vi "Send Generate Event.vi"(8 "Error In":errorcluster, 10 "Event":refnum<class "Event.lvclass">, 11 "Event Source Address":refnum<class "Message Enqueuer.lvclass">) -> (0 "Error Out":errorcluster, 3 "Event Source Address Out":refnum<class "Message Enqueuer.lvclass">)   [LabVIEW 2015, in "Event Source.lvlib" / "Generate Event Msg.lvclass"]
doc: "Send a message to the Event Source Actor to generate the specified event. This method should be called from helper loops within actor core of the Event Source Actor. When the Event Source Actor receives this message he will call Generate Event method.\n\nOnly through calling this method in the helper loops you can be sure all registrants are notified."
uses:
  Generate Event Msg.lvclass
  <vilib>/ActorFramework/Message Enqueuer/Message Enqueuer.lvclass
  Event/Event.lvclass
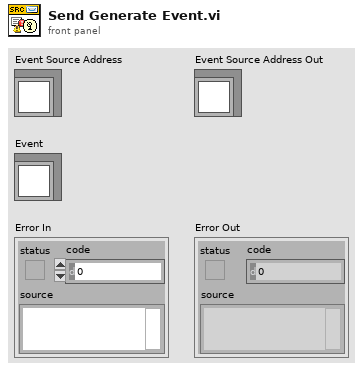
[diagram p1: front panel]
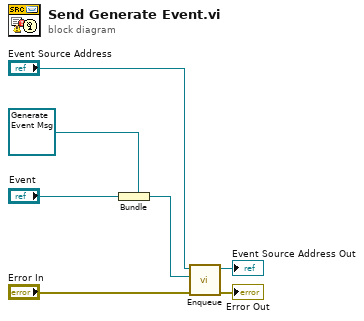
[diagram p0: block diagram]
diagram:
  n1 = Bundle(cluster=refnum<class "Generate Event Msg.lvclass"> refnum ("Message Type"), "Event") -> (w3:refnum<class "Generate Event Msg.lvclass">)
  n2 = call <vilib>:"Enqueue.vi"("error in (no error)"="Error In", "Message"=w3, "Message Enqueuer in"="Event Source Address") -> ("error out"=→"Error Out":errorcluster, "Message Enqueuer out"=→"Event Source Address Out":refnum<class "Message Enqueuer.lvclass">)  [unwired: 7 in]
